vi "p3.1 (hw2).vi"() -> ()   [LabVIEW 2017]
panel:
  out "Green if Random number on red meter is greater":bool
  out "Random number 2":dbl(knob) scale=0.0..1.0
  out "Random number 1":dbl(knob) scale=0.0..1.0
  # "Patrik Sokolowski"
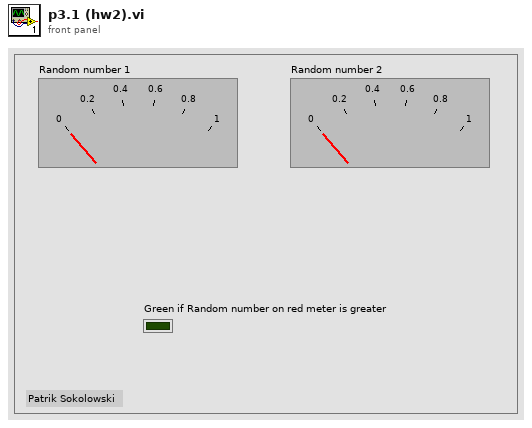
[diagram p1: front panel]
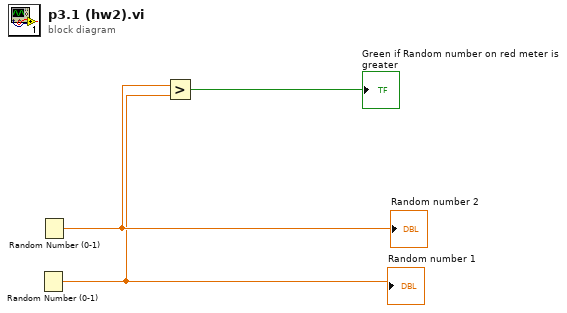
[diagram p0: block diagram]
diagram:
  n1 = Random Number (0-1)() -> (number: 0 to 1=w2:dbl)
  "Random number 1" <- w2
  n2 = Random Number (0-1)() -> (number: 0 to 1=w3:dbl)
  "Random number 2" <- w3
  n3 = Greater?(x=w3, y=w2) -> (0:→"Green if Random number on red meter is greater":bool)
